vi "CircleMask.vi"(6 "y scale":sgl, 7 "Radius Override":bool, 8 "Force radius":dbl, 9 "Array in":i16[][](array[numeric]), 10 "Cursor 1":T1, 11 "Cursor 0":T1) -> (2 "Array 3":i16[][](array[numeric]), 3 "Coordinates":cdb[][](array[numeric]))   [LabVIEW 2022 SP3]
uses:
  <vilib>/Utility/miscctls.llb/LVPointDoubleTypeDef.ctl
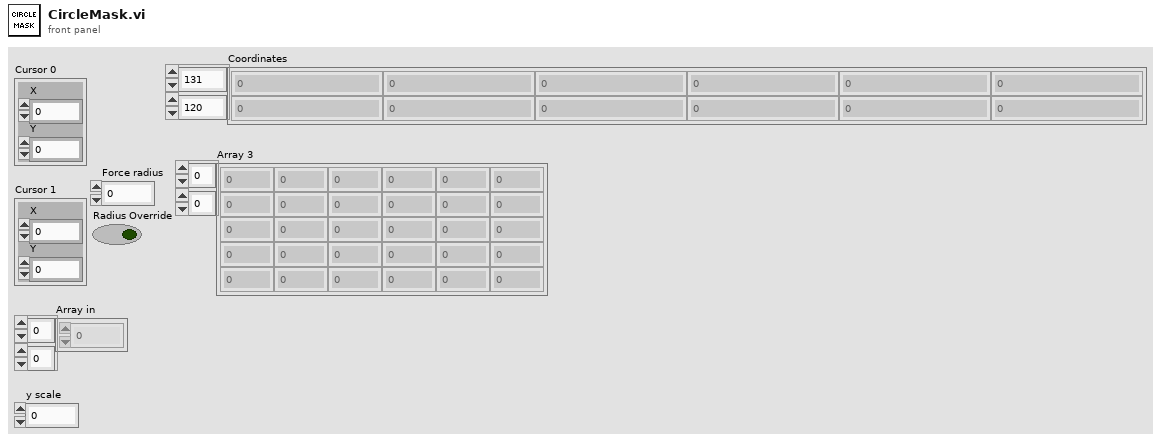
[diagram p1: front panel]
types:
  T1 = typedef "LVPointDoubleTypeDef.ctl" = cluster{"X":dbl, "Y":dbl}
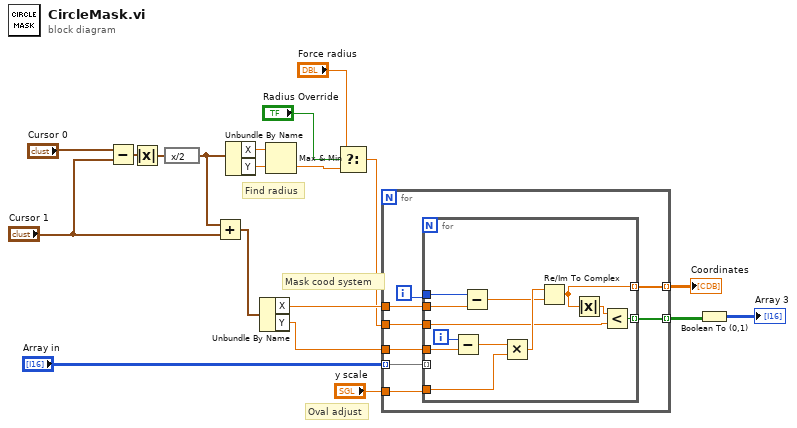
[diagram p0: block diagram]
diagram:
  # "Mask cood system"
  # "Find radius"
  # "Oval adjust"
  n1 = Subtract(x="Cursor 0", y="Cursor 1") -> (x-y=w13:T1)
  n2 = Absolute Value(x=w13) -> (abs(x)=w10:T1)
  n3 = expression code="x/2"(w10) -> (w9:T1)
  n4 = Add(x=w9, y="Cursor 1") -> (x+y=w7:T1)
  n5 = Unbundle By Name(w9) -> ("X"=w12:dbl, "Y"=w11:dbl)
  n6 = Unbundle By Name(w7) -> ("X"=w19:dbl, "Y"=w14:dbl)
  n7 = Max & Min(x=w12, y=w11) -> (min(x,y)=w4:dbl)  [unwired: 1 out]
  n8 = Select(t="Force radius", s="Radius Override", f=w4) -> (s? t:f=w3:dbl)
  n9 = for {
    tunnel: w19 -> [w27]
    tunnel: w14 -> [w25]
    tunnel: [w24] -> w15 mode=indexing
    tunnel: "y scale" -> [w23]
    tunnel: [w22] -> w17 mode=indexing
    tunnel: "Array in" -> [w21] mode=indexing
    tunnel: w3 -> [w20]
    i -> [w26]
    n10 = for {
      tunnel: w27 -> [w37]
      tunnel: w26 -> [w38]
      tunnel: w25 -> [w35]
      tunnel: [w39] -> w24 mode=indexing
      tunnel: w23 -> [w34]
      tunnel: [w31] -> w22 mode=indexing
      tunnel: w21 -> [_] mode=indexing
      tunnel: w20 -> [w28]
      i -> [w36]
      n11 = Subtract(x=w36, y=w35) -> (x-y=w33:dbl)
      n12 = Subtract(x=w38, y=w37) -> (x-y=w29:dbl)
      n13 = Multiply(x=w33, y=w34) -> (x*y=w30:dbl)
      n14 = Re/Im To Complex(1:w29, 2:w30) -> (0:w31:cdb)
      n15 = Absolute Value(x=w31) -> (abs(x)=w32:dbl)
      n16 = Less?(x=w32, y=w28) -> (x < y?=w39:bool)
    }
  }
  "Coordinates" <- w17
  n17 = Boolean To (0,1)(Boolean=w15) -> (0, 1=→"Array 3":i16[][])
